vi "Write Word Log Producer.vi"(8 "error in (no error)":errorcluster, 10 "Communication Bus Template Interfaces:Implementation.lvlib:Logging.lvlib:Word Log Producer.lvclass":refnum<class "Word Log Producer.lvclass">, 11 "Rx Execution Unit in":refnum<class "Rx Execution Unit.lvclass">) -> (0 "error out":errorcluster, 3 "Rx Execution Unit out":refnum<class "Rx Execution Unit.lvclass">)   [LabVIEW 2020, in "Ballard ARINC 429 Engine.lvlib" / "Implementation.lvlib" / "Rx Execution Unit.lvclass"]
uses:
  Rx Execution Unit.lvclass
  Logging/Word Log Producer/Word Log Producer.lvclass
  Rx Execution Unit.lvclass/Rx Execution Unit.ctl
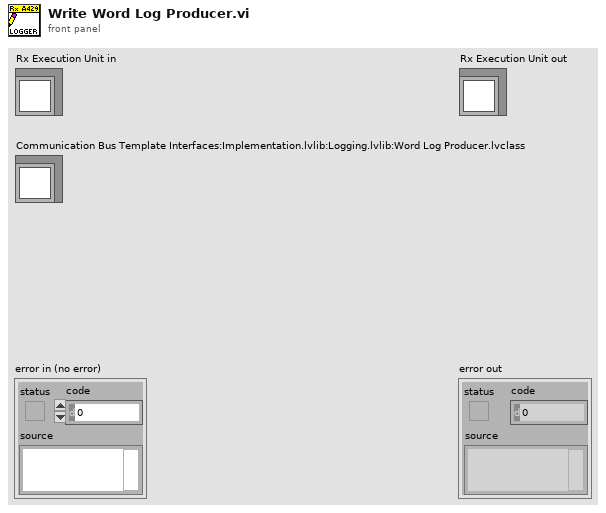
[diagram p1: front panel]
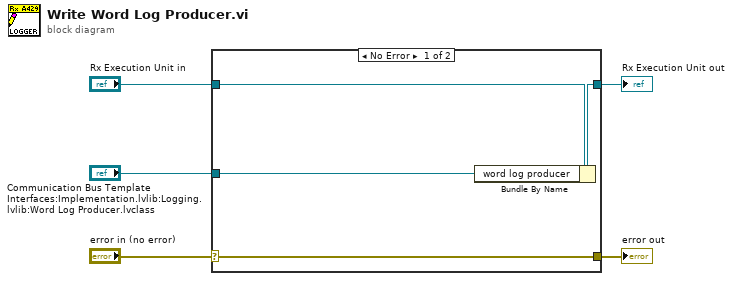
[diagram p0: block diagram]
diagram:
  n1 = case shown="No Error" "error in (no error)" {
    selector: "error in (no error)" -> [w9 w10]
    tunnel: [w9 w10] -> w4
    tunnel: [w7 w11] -> w2
    tunnel: "Rx Execution Unit in" -> [w8 w11]
    tunnel: "Communication Bus Template Interfaces:Implementation.lvlib:Logging.lvlib:Word Log Producer.lvclass" -> [w6 _]
    frame No Error {
      n2 = Bundle By Name(cluster=w8, "word log producer"=w6) -> (w7:refnum<class "Rx Execution Unit.lvclass">)
    }
    frame Error {
    }
  }
  "error out" <- w4
  "Rx Execution Unit out" <- w2
